vi "GetParam.vi"(8 "error in (no error)":errorcluster caption="entrée d'erreur (pas d'erreur)", 11 "HashingVectorizer.lvclass":refnum<class "HashingVectorizer.lvclass">) -> (0 "error out":errorcluster caption="sortie d'erreur", 2 "HashingVectorizer":T1={"encoding"="utf-8", "decode_error"="strict", "strip_accents"="None", "lowercase"=TRUE, "preprocessor"="None", "tokenizer"="None", "stop_words"={"Type"="None", "list"=[]}, "token_pattern"="(?u)\\b\\w\\w+\\b", "ngram_range"={"min_n"=1, "max_n"=1}, "analyzer"="word", "n_features"=1048576, "binary"=FALSE, "norm"="l2", "alternate_sign"=TRUE, "dtype"="float"}, 3 "HashingVectorizer.lvclass":refnum<class "HashingVectorizer.lvclass">)   [LabVIEW 2020, in "HashingVectorizer.lvclass"]
doc: "Get Parameters"
uses:
  HashingVectorizer.lvclass
  HashingVectorizer.lvclass/HashingVectorizer.ctl
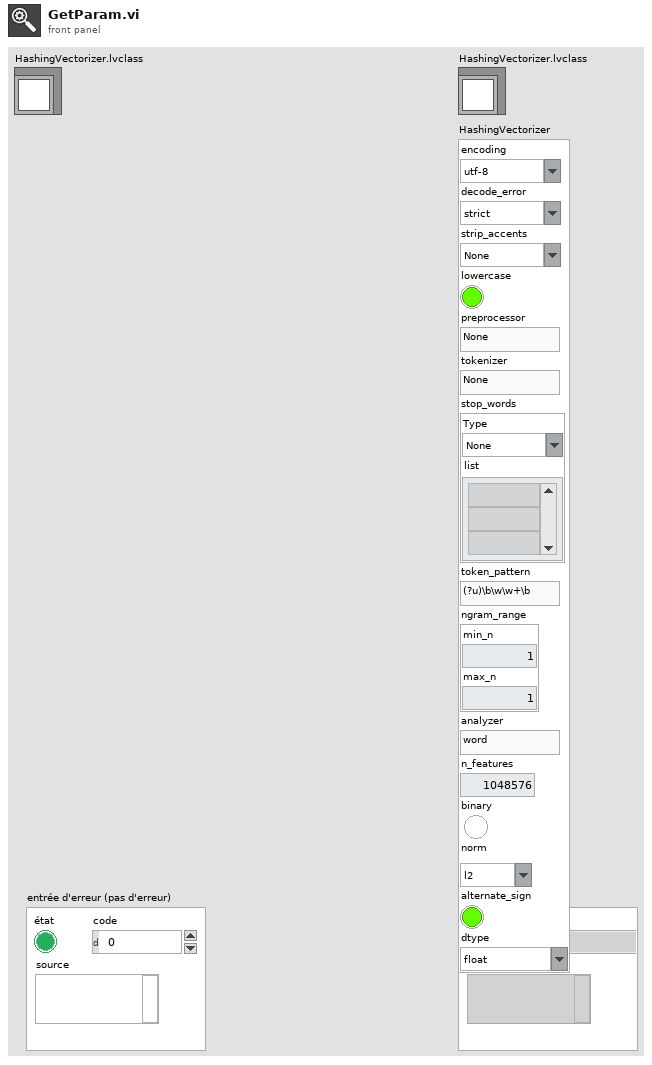
[diagram p1: front panel]
types:
  T1 = cluster{"encoding":string, "decode_error":string, "strip_accents":string, "lowercase":bool, "preprocessor":string, "tokenizer":string, "stop_words":cluster{"Type":string, "list":string[]}, "token_pattern":string, "ngram_range":cluster{"min_n":i32, "max_n":i32}, "analyzer":string, "n_features":i32, "binary":bool, "norm":string, "alternate_sign":bool, "dtype":string}
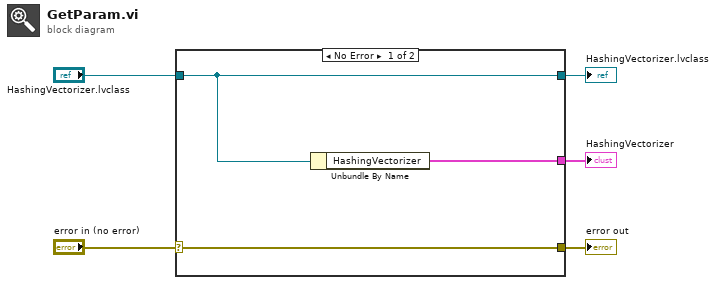
[diagram p0: block diagram]
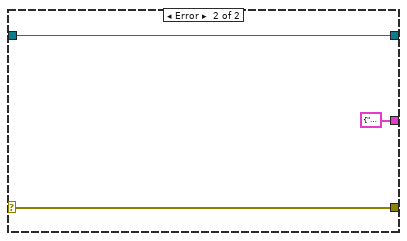
[diagram p2: hidden frame]
diagram:
  n1 = case shown="No Error" "error in (no error)" {
    selector: "error in (no error)" -> [w8 w10]
    tunnel: [w8 w10] -> w4
    tunnel: [w7 w11] -> w2
    tunnel: "HashingVectorizer.lvclass" -> [w7 w11]
    tunnel: [w6 T1 {"encoding"="", "decode_error"="", "strip_accents"="", "lowercase"=FALSE, "preprocessor"="", "tokenizer"="", "stop_words"={"Type"="", "list"=[]}, "token_pattern"="", "ngram_range"={"min_n"=0, "max_n"=0}, "analyzer"="", "n_features"=0, "binary"=FALSE, "norm"="", "alternate_sign"=FALSE, "dtype"=""} ("HashingVectorizer")] -> w1
    frame No Error {
      n2 = Unbundle By Name(w7) -> ("HashingVectorizer"=w6:T1)
    }
    frame Error {
    }
  }
  "error out" <- w4
  "HashingVectorizer.lvclass" <- w2
  "HashingVectorizer" <- w1
